vi "SRingLastRead.vi"(1 "pixel":u32=600) -> (0 "Data Values":u16[](graph))   [LabVIEW 2015]
uses:
  ESLSCDLL.dll
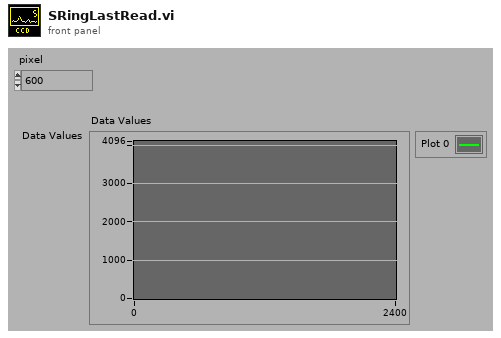
[diagram p1: front panel]
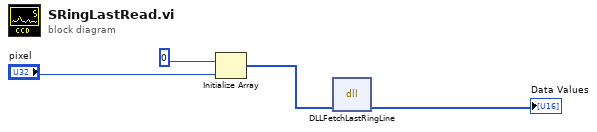
[diagram p0: block diagram]
diagram:
  n1 = Initialize Array(u32 0, "pixel") -> (w2:u32[])
  n2 = dll-call lib="C:/ENTW/PCIE/64bit/lv64/1cam/board.vis/ESLSCDLL.dll" fn="DLLFetchLastRingLine"("dioden"=w2) -> ("dioden"=→"Data Values":u16[])  [unwired: 4 in, 2 out]
